vi "rqcAlice SPI PM Level test.vi"() -> ()   [LabVIEW 2018]
uses:
  <vilib>/Platform/TimedLoop/XDataNode/timing_clust.ctl
  <vilib>/Platform/TimedLoop/XDataNode/nitl_modes.ctl
  <vilib>/Platform/TimedLoop/XDataNode/wakeup.ctl
  <vilib>/rvi/Emulation/niFpgaSctlEmulationGetInTimedLoop.vi
  <vilib>/rvi/Emulation/niFpgaEmulationReportErrorSimple.vi
  <vilib>/rvi/Emulation/niFpgaGetClockAttributes.vi
  <vilib>/rvi/Emulation/niFpgaCriticalErrorInLSC.vi
  <vilib>/rvi/eio/common/nirviEmuTemplateMethod_errors.vi
  <vilib>/Platform/TimedLoop/XDataNode/XDataNode.xnode
  <vilib>/eio/EIONode/EIONode.xnode
  <vilib>/Platform/TimedLoop/XDataNode/XDNodeRunTimeDep.lvlib
panel:
  in  "send clock":bool
  in  "level":u8
  in  "SPI.data":u32 format="%024b"
  in  "SPI.write":bool
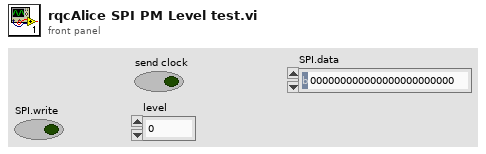
[diagram p1: front panel]
types:
  T1 = typedef "XDNodeRunTimeDep.lvlib/timing_clust.ctl" = cluster{"Expected End [f-1]":u64, "Actual End [f-1]":u64, "Finished Late? [f-1]":bool, "Expected End [i-1]":u64, "Actual End [i-1]":u64, "Finished Late? [i-1]":bool, "Expected Start [i]":u64, "Actual Start [i]":u64, "Expected Start [f]":u64, "Actual Start [f]":u64, "Source Name":string, "Structure Name":string, "Period":i64, "Deadline":i64, "Offset":i64, "Start":i64, "Priority":i32, "Timeout":i32, "Mode":T2, "Wakeup Reason":T3, "Error":errorcluster, "Source Type":string, "Secondary Source Type":string, "Global End Time":u64, "Global Start Time":u64, "Frame Duration":u64, "Iteration Duration":u64, "Assigned CPU":i32, "I/O Scan Engine Mode":u32}
  T2 = typedef "XDNodeRunTimeDep.lvlib/nitl_modes.ctl" = enum32{"No Change", "Process missed periods, maintain original phase", "Discard missed periods, maintain original phase", "Process missed periods, ignore original phase", "Discard missed periods, ignore original phase"}
  T3 = typedef "XDNodeRunTimeDep.lvlib/wakeup.ctl" = enum32{"Normal", "Aborted", "Asynchronous wakeup", "Timing source error", "Timed loop error", "Timeout"}
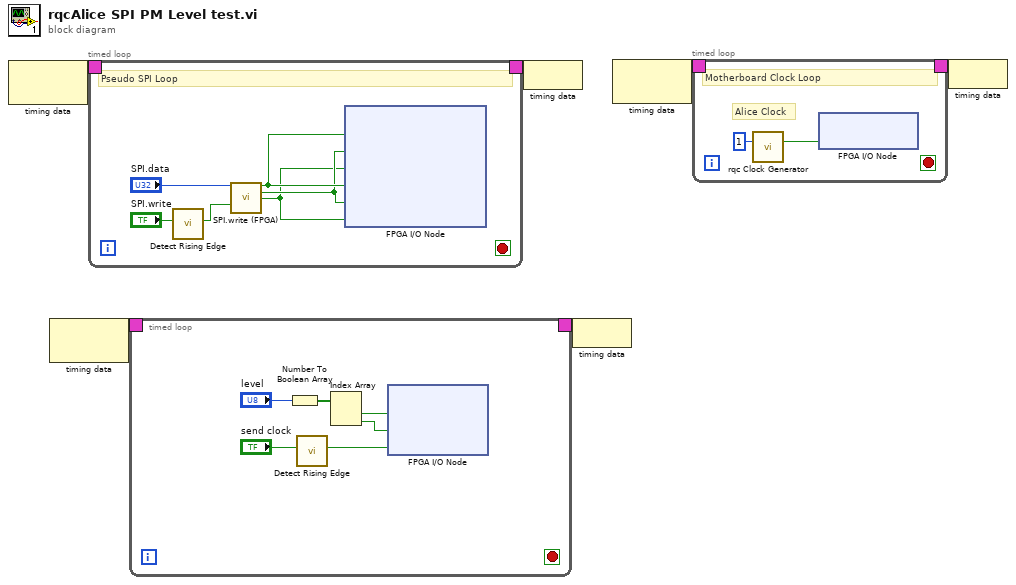
[diagram p0: block diagram]
diagram:
  n1 = node-c288() -> (w6:T1)  [unwired: 1 in]
  n2 = node-c288() -> (w4:T1)  [unwired: 1 in]
  n3 = timed-loop {
    timing: w6 -> [_]
    timing-out: [_] -> w5
    stop <- _ stop-if-true
    # "Pseudo SPI Loop"
    n4 = call <vilib>:"Detect Rising Edge.vi"("signal"="SPI.write") -> ("edge detected"=w7:bool)  [unwired: 10 in]
    n5 = call "SPI.write (FPGA).vi"("data in"="SPI.data", "write"=w7) -> ("data"=w11:bool, "we"=w10:bool, "clk"=w9:bool)  [unwired: 11 in]
    n6 = xnode "FPGA I/O Node"("SPI/DATA (service)"=w11, "SPI/EN (service)"=w10, "SPI/CLK (service)"=w9, "SPI/Data"=w11, "SPI/EN"=w10, "SPI/CLK"=w9) -> ()  [unwired: 6 in, 6 out]
  }
  n7 = timed-loop {
    timing: w4 -> [_]
    timing-out: [_] -> w3
    stop <- _ stop-if-true
    n8 = Number To Boolean Array(number="level") -> (Boolean array=w20:bool[])
    n9 = call <vilib>:"Detect Rising Edge.vi"("signal"="send clock") -> ("edge detected"=w17:bool)  [unwired: 10 in]
    n10 = Index Array(array=w20) -> (element #1=w19:bool, element #2=w18:bool)  [unwired: 2 in]
    n11 = xnode "FPGA I/O Node"("DAC/bit2"=w19, "DAC/bit3"=w18, "DAC/clock"=w17) -> ()  [unwired: 3 in, 3 out]
  }
  n12 = node-c288(w5) -> ()
  n13 = node-c288(w3) -> ()
  n14 = node-c288() -> (w2:T1)  [unwired: 1 in]
  n15 = timed-loop {
    timing: w2 -> [_]
    timing-out: [_] -> w1
    stop <- _ stop-if-true
    # "Alice Clock"
    # "Motherboard Clock Loop"
    n16 = call "rqc Clock Generator.vi"("SCTL clock devider"=u8 1) -> ("clock out"=w23:bool)  [unwired: 14 in]
    n17 = xnode "FPGA I/O Node"("AliceClock"=w23) -> ()  [unwired: 1 in, 1 out]
  }
  n18 = node-c288(w1) -> ()
